vi "Clear FPGA.vi"(8 "error in (no error)":errorcluster, 11 "Item Ref in":T1 format="%.0x") -> (0 "error out":errorcluster, 3 "Item Ref out":T1 format="%.0x")   [LabVIEW 2016, in "Scan Engine Custom Device.lvlib"]
uses:
  Scan Engine Custom Device.lvlib
  <vilib>/NI Veristand/Custom Device API/Custom Device Item Ref.ctl
  <vilib>/NI Veristand/Custom Device API/Custom Device API.lvlib
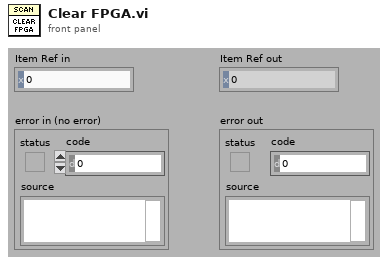
[diagram p1: front panel]
types:
  T1 = typedef "Custom Device API.lvlib/Custom Device Item Ref.ctl" = u64
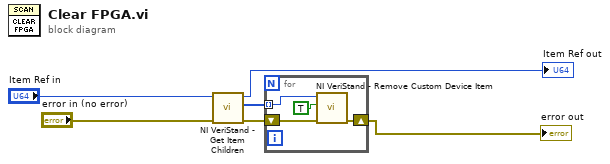
[diagram p0: block diagram]
diagram:
  n1 = call <vilib>:"NI VeriStand - Get Item Children.vi"("error in (no error)"="error in (no error)", "Item Ref in"="Item Ref in") -> ("error out"=w6:errorcluster, "Child Refs"=w5:T1[], "Item Ref out"=→"Item Ref out":T1)  [unwired: 6 in, 1 out]
  n2 = for {
    shift-right: [w7] -> w2
    shift-left: w6 -> [w10]
    tunnel: w5 -> [w9] mode=indexing
    n3 = call <vilib>:"NI VeriStand - Remove Custom Device Item.vi"("error in (no error)"=w10, "Force Delete (F)"=TRUE, "Item Ref in"=w9) -> ("error out"=w7:errorcluster)  [unwired: 7 in, 1 out]
  }
  "error out" <- w2
